vi "Get LabVIEW File Format Version.vi"(8 "error in (no error)":errorcluster, 11 "VI Path":path) -> (0 "error out":errorcluster, 2 "Version Number":u32, 3 "Get VI:Version":string)   [LabVIEW 2020]
doc: "Returns the LabVIEW file format version of the VI."
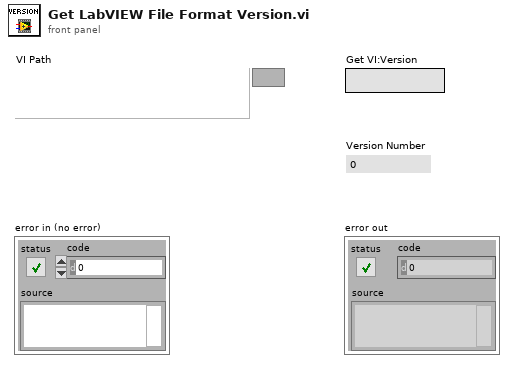
[diagram p1: front panel]
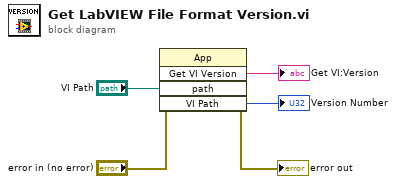
[diagram p0: block diagram]
diagram:
  n1 = invoke class="App" method="Get VI Version"(error in="error in (no error)", "path"="VI Path") -> (error out=→"error out":errorcluster, "GetVIVers"=→"Get VI:Version":string, "VI Path"=→"Version Number":u32)  [unwired: 3 in, 2 out]
